vi "Gas_Commands.vi"(1 "Debug Mode":bool, 2 "Flow Array":dbl[](array[numeric]), 3 "Argument List":string[](array[string]), 4 "Command":string) -> ()   [LabVIEW 2011]
doc: "This VI will utilize the supplied arguments to set the corresponding relays of the MOCVD system for the gas given by the \"Command\" parameter. For example, if the strings \"Active\" and \"Bubbler\" are present in the \"Argument List\", the \"Active\" and \"Bubbler\" relays will be enabled for the given gas. This VI also sets the flows given by the \"Flow Array\" parameter, with indicies 0, 1, 2, and 3 corresponding to Flows 1, 2, 3, and 4 for the given gas. The \"Debug\" parameter disables all hardware communications."
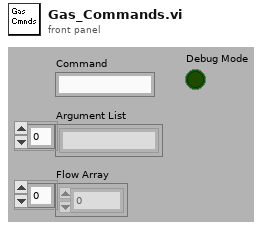
[diagram p1: front panel]
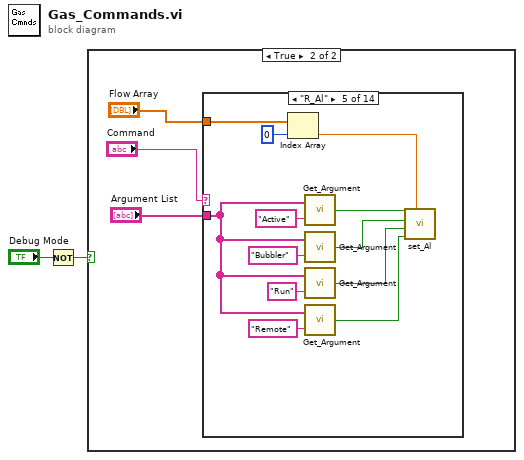
[diagram p0: block diagram]
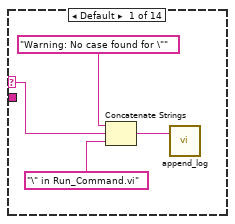
[diagram p3: hidden frame]
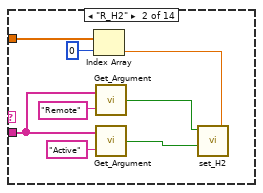
[diagram p4: hidden frame]
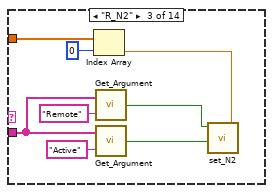
[diagram p5: hidden frame]
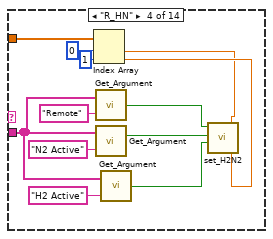
[diagram p6: hidden frame]
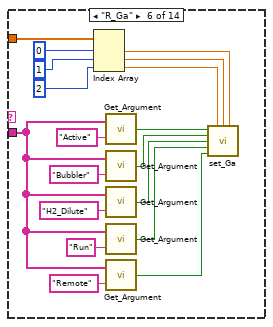
[diagram p7: hidden frame]
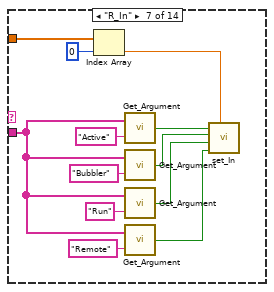
[diagram p8: hidden frame]
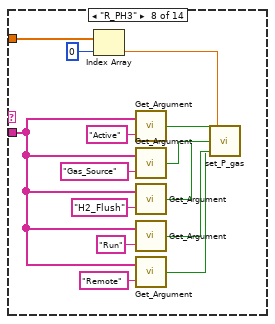
[diagram p9: hidden frame]
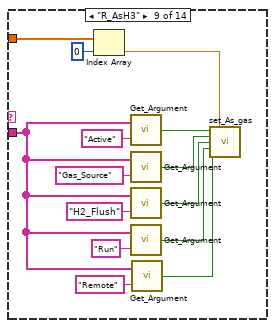
[diagram p10: hidden frame]
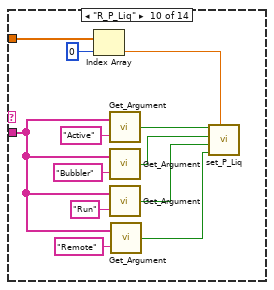
[diagram p11: hidden frame]
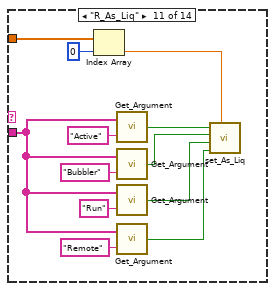
[diagram p12: hidden frame]
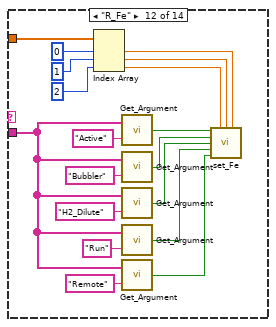
[diagram p13: hidden frame]
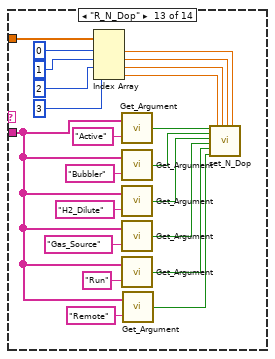
[diagram p14: hidden frame]
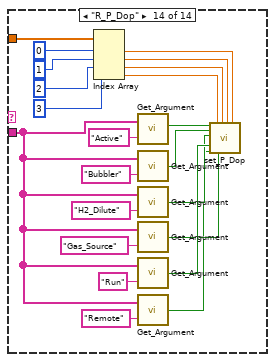
[diagram p15: hidden frame]
diagram:
  n1 = Not(x="Debug Mode") -> (.not. x?=w2:bool)
  n2 = case shown="True" w2 {
    frame False {
    }
    frame True {
      n3 = case shown="\"R_Al\"" "Command" {
        selector: "Command" -> [w8 _ _ _ _ _ _ _ _ _ _ _ _ _]
        tunnel: "Argument List" -> [_ w11 w19 w29 w39 w51 w69 w81 w97 w109 w121 w133 w151 w173]
        tunnel: "Flow Array" -> [_ w16 w24 w36 w46 w59 w76 w89 w103 w116 w128 w145 w167 w189]
        frame Default {
          n4 = Concatenate Strings("Warning: No case found for \"" ("message"), w8, "\" in Run_Command.vi" ("string")) -> (w6:string)
          n5 = call "append_log.vi"("New Log String"=w6) -> ()  [unwired: 1 in, 1 out]
        }
        frame "R_H2" {
          n6 = Index Array(array=w16, index=0) -> (element=w14:dbl)
          n7 = call "Get_Argument.vi"("Argument"="Remote", "Argument List"=w11) -> ("Enabled"=w10:bool)
          n8 = call "Get_Argument.vi"("Argument"="Active", "Argument List"=w11) -> ("Enabled"=w13:bool)
          n9 = call "set_H2.vi"("Manifold H2 Flow"=w14, "H2 Active"=w13, "Remote"=w10) -> ()  [unwired: 3 in]
        }
        frame "R_N2" {
          n10 = Index Array(array=w24, index=0) -> (element=w21:dbl)
          n11 = call "Get_Argument.vi"("Argument"="Remote", "Argument List"=w19) -> ("Enabled"=w18:bool)
          n12 = call "Get_Argument.vi"("Argument"="Active", "Argument List"=w19) -> ("Enabled"=w22:bool)
          n13 = call "set_N2.vi"("Manifold N2 Flow"=w21, "N2 Active"=w22, "Remote"=w18) -> ()  [unwired: 3 in]
        }
        frame "R_HN" {
          n14 = Index Array(array=w36, index #1=0 ("index"), index #2=1 ("index")) -> (element #1=w26:dbl, element #2=w27:dbl)
          n15 = call "Get_Argument.vi"("Argument"="Remote", "Argument List"=w29) -> ("Enabled"=w33:bool)
          n16 = call "Get_Argument.vi"("Argument"="N2 Active", "Argument List"=w29) -> ("Enabled"=w32:bool)
          n17 = call "Get_Argument.vi"("Argument"="H2 Active", "Argument List"=w29) -> ("Enabled"=w31:bool)
          n18 = call "set_H2N2.vi"("Manifold N2 Flow"=w27, "Manifold H2 Flow"=w26, "H2 Active"=w31, "N2 Active"=w32, "Remote"=w33) -> ()  [unwired: 1 in]
        }
        frame "R_Al" {
          n19 = Index Array(array=w46, index=0) -> (element=w44:dbl)
          n20 = call "Get_Argument.vi"("Argument"="Active", "Argument List"=w39) -> ("Enabled"=w43:bool)
          n21 = call "Get_Argument.vi"("Argument"="Bubbler", "Argument List"=w39) -> ("Enabled"=w42:bool)
          n22 = call "Get_Argument.vi"("Argument"="Run", "Argument List"=w39) -> ("Enabled"=w41:bool)
          n23 = call "Get_Argument.vi"("Argument"="Remote", "Argument List"=w39) -> ("Enabled"=w38:bool)
          n24 = call "set_Al.vi"("ALMFC1"=w44, "Remote"=w38, "Run"=w41, "Bubbler In"=w42, "Active"=w43) -> ()  [unwired: 5 out]
        }
        frame "R_Ga" {
          n25 = Index Array(array=w59, index #1=0 ("index"), index #2=1 ("index"), index #3=2 ("index")) -> (element #1=w55:dbl, element #2=w54:dbl, element #3=w53:dbl)
          n26 = call "Get_Argument.vi"("Argument"="Active", "Argument List"=w51) -> ("Enabled"=w66:bool)
          n27 = call "Get_Argument.vi"("Argument"="Bubbler", "Argument List"=w51) -> ("Enabled"=w64:bool)
          n28 = call "Get_Argument.vi"("Argument"="H2_Dilute", "Argument List"=w51) -> ("Enabled"=w62:bool)
          n29 = call "Get_Argument.vi"("Argument"="Run", "Argument List"=w51) -> ("Enabled"=w60:bool)
          n30 = call "Get_Argument.vi"("Argument"="Remote", "Argument List"=w51) -> ("Enabled"=w50:bool)
          n31 = call "set_Ga.vi"("Active"=w66, "GAMFC3"=w53, "GAMFC2"=w54, "GAMFC1"=w55, "Bubbler In"=w64, "H2 Dilute"=w62, "Run"=w60, "Remote"=w50) -> ()  [unwired: 8 out]
        }
        frame "R_In" {
          n32 = Index Array(array=w76, index=0) -> (element=w71:dbl)
          n33 = call "Get_Argument.vi"("Argument"="Active", "Argument List"=w69) -> ("Enabled"=w72:bool)
          n34 = call "Get_Argument.vi"("Argument"="Bubbler", "Argument List"=w69) -> ("Enabled"=w73:bool)
          n35 = call "Get_Argument.vi"("Argument"="Run", "Argument List"=w69) -> ("Enabled"=w74:bool)
          n36 = call "Get_Argument.vi"("Argument"="Remote", "Argument List"=w69) -> ("Enabled"=w68:bool)
          n37 = call "set_In.vi"("INMFC1"=w71, "Remote"=w68, "Run"=w74, "Bubbler In"=w73, "Active"=w72) -> ()  [unwired: 5 out]
        }
        frame "R_PH3" {
          n38 = Index Array(array=w89, index=0) -> (element=w87:dbl)
          n39 = call "Get_Argument.vi"("Argument"="Active", "Argument List"=w81) -> ("Enabled"=w86:bool)
          n40 = call "Get_Argument.vi"("Argument"="Gas_Source", "Argument List"=w81) -> ("Enabled"=w85:bool)
          n41 = call "Get_Argument.vi"("Argument"="H2_Flush", "Argument List"=w81) -> ("Enabled"=w84:bool)
          n42 = call "Get_Argument.vi"("Argument"="Run", "Argument List"=w81) -> ("Enabled"=w83:bool)
          n43 = call "Get_Argument.vi"("Argument"="Remote", "Argument List"=w81) -> ("Enabled"=w80:bool)
          n44 = call "set_P_gas.vi"("Run"=w83, "Gas In"=w85, "Active"=w86, "P_Gas Remote"=w80, "H2 Flush"=w84, "P_Gas Flow"=w87) -> ()
        }
        frame "R_AsH3" {
          n45 = Index Array(array=w103, index=0) -> (element=w101:dbl)
          n46 = call "Get_Argument.vi"("Argument"="Active", "Argument List"=w97) -> ("Enabled"=w100:bool)
          n47 = call "Get_Argument.vi"("Argument"="Gas_Source", "Argument List"=w97) -> ("Enabled"=w99:bool)
          n48 = call "Get_Argument.vi"("Argument"="H2_Flush", "Argument List"=w97) -> ("Enabled"=w94:bool)
          n49 = call "Get_Argument.vi"("Argument"="Run", "Argument List"=w97) -> ("Enabled"=w95:bool)
          n50 = call "Get_Argument.vi"("Argument"="Remote", "Argument List"=w97) -> ("Enabled"=w96:bool)
          n51 = call "set_As_gas.vi"("Active"=w100, "As_Gas Flow"=w101, "Gas In"=w99, "H2 Flush"=w94, "Run"=w95, "Remote"=w96) -> ()  [unwired: 10 out]
        }
        frame "R_P_Liq" {
          n52 = Index Array(array=w116, index=0) -> (element=w114:dbl)
          n53 = call "Get_Argument.vi"("Argument"="Active", "Argument List"=w109) -> ("Enabled"=w111:bool)
          n54 = call "Get_Argument.vi"("Argument"="Bubbler", "Argument List"=w109) -> ("Enabled"=w112:bool)
          n55 = call "Get_Argument.vi"("Argument"="Run", "Argument List"=w109) -> ("Enabled"=w113:bool)
          n56 = call "Get_Argument.vi"("Argument"="Remote", "Argument List"=w109) -> ("Enabled"=w108:bool)
          n57 = call "set_P_Liq.vi"("flow 1"=w114, "Remote"=w108, "Run"=w113, "Bubbler In"=w112, "Active"=w111) -> ()  [unwired: 5 in]
        }
        frame "R_As_Liq" {
          n58 = Index Array(array=w128, index=0) -> (element=w123:dbl)
          n59 = call "Get_Argument.vi"("Argument"="Active", "Argument List"=w121) -> ("Enabled"=w124:bool)
          n60 = call "Get_Argument.vi"("Argument"="Bubbler", "Argument List"=w121) -> ("Enabled"=w125:bool)
          n61 = call "Get_Argument.vi"("Argument"="Run", "Argument List"=w121) -> ("Enabled"=w126:bool)
          n62 = call "Get_Argument.vi"("Argument"="Remote", "Argument List"=w121) -> ("Enabled"=w120:bool)
          n63 = call "set_As_Liq.vi"("ASLMFC1"=w123, "Remote"=w120, "Run"=w126, "Bubbler In"=w125, "Active"=w124) -> ()  [unwired: 5 in]
        }
        frame "R_Fe" {
          n64 = Index Array(array=w145, index #1=0 ("index"), index #2=1 ("index"), index #3=2 ("index")) -> (element #1=w137:dbl, element #2=w136:dbl, element #3=w135:dbl)
          n65 = call "Get_Argument.vi"("Argument"="Active", "Argument List"=w133) -> ("Enabled"=w142:bool)
          n66 = call "Get_Argument.vi"("Argument"="Bubbler", "Argument List"=w133) -> ("Enabled"=w141:bool)
          n67 = call "Get_Argument.vi"("Argument"="H2_Dilute", "Argument List"=w133) -> ("Enabled"=w140:bool)
          n68 = call "Get_Argument.vi"("Argument"="Run", "Argument List"=w133) -> ("Enabled"=w143:bool)
          n69 = call "Get_Argument.vi"("Argument"="Remote", "Argument List"=w133) -> ("Enabled"=w132:bool)
          n70 = call "set_Fe.vi"("Active"=w142, "Fe Flow 3"=w135, "Fe Flow 2"=w136, "Fe Flow 1"=w137, "Bubbler"=w141, "H2 Dilute"=w140, "Run"=w143, "Remote"=w132) -> ()  [unwired: 8 out]
        }
        frame "R_N_Dop" {
          n71 = Index Array(array=w167, index #1=0 ("index"), index #2=1 ("index"), index #3=2 ("index"), index #4=3 ("index")) -> (element #1=w162:dbl, element #2=w161:dbl, element #3=w160:dbl, element #4=w159:dbl)
          n72 = call "Get_Argument.vi"("Argument"="Active", "Argument List"=w151) -> ("Enabled"=w158:bool)
          n73 = call "Get_Argument.vi"("Argument"="Bubbler", "Argument List"=w151) -> ("Enabled"=w157:bool)
          n74 = call "Get_Argument.vi"("Argument"="H2_Dilute", "Argument List"=w151) -> ("Enabled"=w153:bool)
          n75 = call "Get_Argument.vi"("Argument"="Gas_Source", "Argument List"=w151) -> ("Enabled"=w154:bool)
          n76 = call "Get_Argument.vi"("Argument"="Run", "Argument List"=w151) -> ("Enabled"=w156:bool)
          n77 = call "Get_Argument.vi"("Argument"="Remote", "Argument List"=w151) -> ("Enabled"=w150:bool)
          n78 = call "set_N_Dop.vi"("Active"=w158, "Bubbler In"=w157, "H2 Dilute"=w153, "Gas Source In"=w154, "Run"=w156, "Remote"=w150, "Gas Flow"=w159, "Flow 3"=w160, "Flow 2"=w161, "Flow 1"=w162) -> ()  [unwired: 10 out]
        }
        frame "R_P_Dop" {
          n79 = Index Array(array=w189, index #1=0 ("index"), index #2=1 ("index"), index #3=2 ("index"), index #4=3 ("index")) -> (element #1=w178:dbl, element #2=w177:dbl, element #3=w176:dbl, element #4=w175:dbl)
          n80 = call "Get_Argument.vi"("Argument"="Active", "Argument List"=w173) -> ("Enabled"=w183:bool)
          n81 = call "Get_Argument.vi"("Argument"="Bubbler", "Argument List"=w173) -> ("Enabled"=w179:bool)
          n82 = call "Get_Argument.vi"("Argument"="H2_Dilute", "Argument List"=w173) -> ("Enabled"=w180:bool)
          n83 = call "Get_Argument.vi"("Argument"="Gas_Source", "Argument List"=w173) -> ("Enabled"=w181:bool)
          n84 = call "Get_Argument.vi"("Argument"="Run", "Argument List"=w173) -> ("Enabled"=w182:bool)
          n85 = call "Get_Argument.vi"("Argument"="Remote", "Argument List"=w173) -> ("Enabled"=w172:bool)
          n86 = call "set_P_Dop.vi"("P_Dop Active"=w183, "P_Dop Bubbler"=w179, "P_Dop H2 Dilute"=w180, "P_Dop Gas Source"=w181, "P_Dop Run"=w182, "P_Dop Remote"=w172, "P_Dop Flow 4"=w175, "P_Dop Flow 3"=w176, "P_Dop Flow 2"=w177, "P_Dop Flow 1"=w178) -> ()  [unwired: 10 out]
        }
      }
    }
  }
